vi "Refresh Request.vi"(9 "Refresh Token":string, 10 "Client":refnum<class "Client.lvclass">, 11 "Request in":refnum<class "Request.lvclass">) -> (2 "POST Buffer":string, 3 "Request URL":string)   [LabVIEW 2020, in "OAuth2.lvlib" / "Request.lvclass"]
uses:
  Request.lvclass
  Request.lvclass/Request.ctl
  HTTP Utils/HTTP Utils.lvlib
  Client/Client.lvclass
  <vilib>/IlluminatedG/lv-stream/URI/URI.lvclass
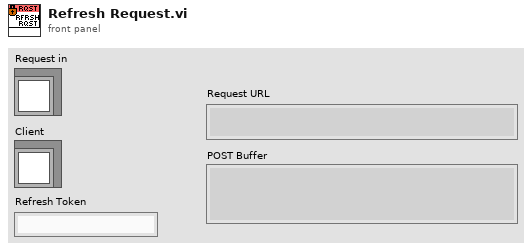
[diagram p1: front panel]
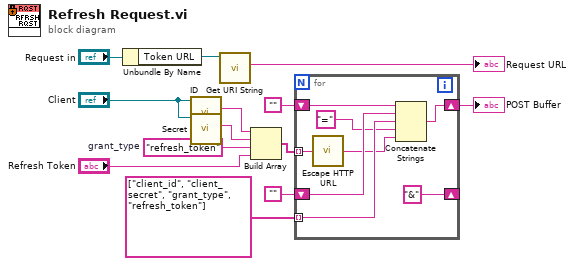
[diagram p0: block diagram]
diagram:
  w2 = "refresh_token"  # grant_type
  n1 = Unbundle By Name("Request in") -> ("Token URL"=w13:refnum<class "URI.lvclass">)
  n2 = call "ID.vi"("Client in"="Client") -> ("Client ID"=w4:string)  [unwired: 10 in]
  n3 = call "Secret.vi"("Client in"="Client") -> ("Client Secret"=w3:string)  [unwired: 10 in]
  n4 = call <vilib>:"Get URI String.vi"("URI in"=w13) -> ("URI String"=→"Request URL":string)  [unwired: 8 in, 2 out]
  n5 = Build Array(w4, w3, w2, "Refresh Token") -> (w7:string[])
  n6 = for {
    tunnel: w7 -> [w21] mode=indexing
    tunnel: string[] ["client_id", "client_secret", "grant_type", "refresh_token"] -> [w17] mode=indexing
    shift-right: ["&"] -> _
    shift-left: "" -> [w18]
    shift-right: [w14] -> w9
    shift-left: "" -> [w19]
    n7 = call "Escape HTTP URL.vi"("unescaped string in"=w21) -> ("escaped string out"=w15:string)
    n8 = Concatenate Strings(w19, w18, w17, "=" ("string"), w15) -> (w14:string)
  }
  "POST Buffer" <- w9
